vi "PickPlaceAccuracy.vi"() -> ()   [LabVIEW 2019]
panel:
  in  "GoToPlateHB":string="G1 X1143.6066027 Y1005.0612551 F100\rG1 Z64.7125267"
  in  "MatchParameters":T1={"Number of Matches Requested"=1, "Minimum Match Score"=950.0, "Angle Ranges"=[{"Start Angle"=0.0, "End Angle"=0.0}]}
  in  "AtPlate":bool
  in  "SafeMaxZAssembly":dbl=70.0 format="%#_13g"
  in  "Assembly_XYZU":string="G1 X218.5881767 Y999.2858584 F100\rG1 Z67.8627861"
  out "error out":errorcluster
  out "Plate_XYZU":string
  in  "TemplateFileName":string
  out "Image":T2(plugin-control)
  in  "Tolerance":dbl=0.005 format="%#_13g"
  in  "InitialStepSize":dbl=0.1
  in  "SafeMaxZPlate":dbl=77.0 format="%#_13g"
  in  "GoToPlateSi":string="G1 X844.5335768 Y1006.4997118 F100\rG1 Z74.2865084"
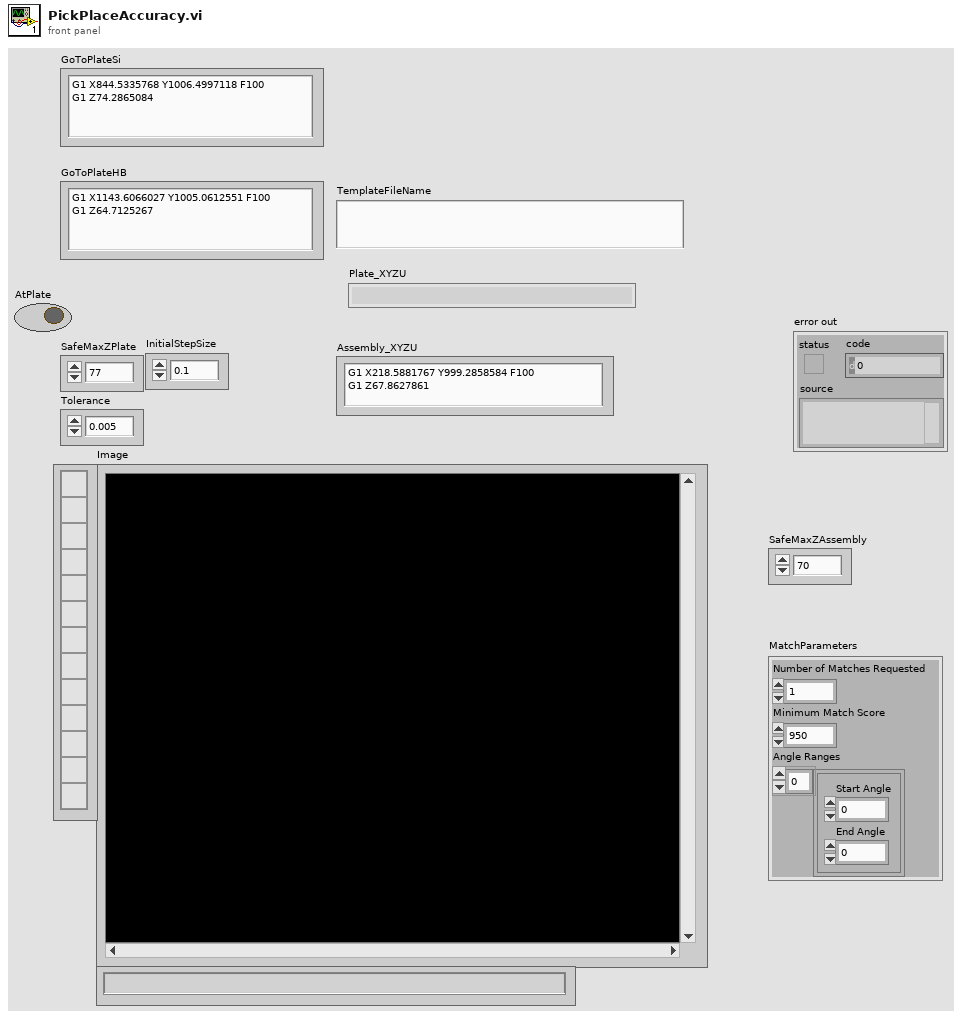
[diagram p1: front panel]
types:
  T1 = cluster{"Number of Matches Requested":i32, "Minimum Match Score":sgl, "Angle Ranges":cluster{"Start Angle":sgl, "End Angle":sgl}[]}
  T2 = typedef "IMAQ Image.ctl" = refnum<image>
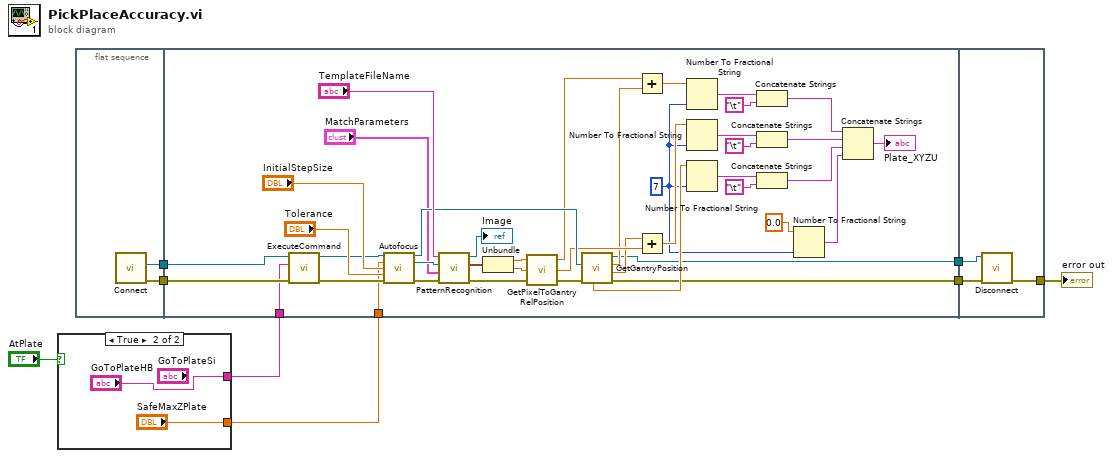
[diagram p0: block diagram]
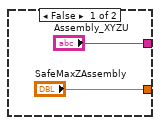
[diagram p2: hidden frame]
diagram:
  n1 = case shown="True" "AtPlate" {
    tunnel: ["Assembly_XYZU" "GoToPlateHB"] -> w4
    tunnel: ["SafeMaxZAssembly" "SafeMaxZPlate"] -> w3
    frame False {
    }
    frame True {
    }
  }
  n2 = flat-sequence {
    tunnel: [w14] -> w8
    tunnel: [w13] -> w6
    tunnel: w8 -> [w54]
    tunnel: w6 -> [w55]
    tunnel: w4 -> [w20]
    tunnel: w3 -> [w19]
    tunnel: [w18] -> w2
    tunnel: [w17] -> w1
    tunnel: [w58] -> w7
    tunnel: w2 -> [w57]
    tunnel: w1 -> [w56]
    frame #0 {
      n3 = call "Connect.vi"() -> ("error out"=w13:errorcluster, "controller"=w14:refnum<k24>)  [unwired: 10 in]
    }
    frame #1 {
      w33 = i16 7 ("precision (6)")
      n4 = call "ExecuteCommand.vi"("error in (no error)"=w55, "Command Code"=w20, "controller in"=w54) -> ("error out"=w21:errorcluster, "controller out"=w22:refnum<k24>)  [unwired: 6 in, 1 out]
      n5 = call "Autofocus.vi"("controller in"=w22, "SafeMaxZ"=w19, "InitialStepSize"="InitialStepSize", "Tolerance"="Tolerance", "error in (no error)"=w21) -> ("controller out"=w50:refnum<k24>, "Image"=w24:T2, "error out"=w29:errorcluster)  [unwired: 6 in, 2 out]
      n6 = call "PatternRecognition.vi"("error in (no error)"=w29, "MatchParameters"="MatchParameters", "ImageIn"=w24, "TemplateFileName"="TemplateFileName") -> ("error out"=w25:errorcluster, "Position"=w28:cluster{"x":sgl, "y":sgl}, "ImageFoundPattern"=→"Image":T2)  [unwired: 2 in, 2 out]
      n7 = Unbundle(w28) -> ("x"=w27:sgl, "y"=w26:sgl)
      n8 = call "GetPixelToGantryRelPosition.vi"("error in (no error)"=w25, "PixelY"=w26, "PixelX"=w27) -> ("error out"=w47:errorcluster, "YmmRelGH"=w48:dbl, "XmmRelGH"=w49:dbl)
      n9 = call "GetGantryPosition.vi"("error in (no error)"=w47, "Controller In"=w50) -> ("error out"=w18:errorcluster, "Position Y"=w36:dbl, "Position X"=w35:dbl, "controller out"=w17:refnum<k24>, "Position Z"=w44:dbl)  [unwired: 3 in, 2 out]
      n10 = Add(x=w49, y=w35) -> (x+y=w42:dbl)
      n11 = Add(x=w36, y=w48) -> (x+y=w43:dbl)
      n12 = Number To Fractional String(number=w42, precision (6)=w33) -> (F-format string=w37:string)  [unwired: 2 in]
      n13 = Number To Fractional String(number=w43, precision (6)=w33) -> (F-format string=w38:string)  [unwired: 2 in]
      n14 = Number To Fractional String(number=w44, precision (6)=w33) -> (F-format string=w45:string)  [unwired: 2 in]
      n15 = Concatenate Strings(w37, "\t") -> (w39:string)
      n16 = Concatenate Strings(w38, "\t") -> (w40:string)
      n17 = Concatenate Strings(w45, "\t") -> (w46:string)
      n18 = Number To Fractional String(number=0.0, precision (6)=w33) -> (F-format string=w16:string)  [unwired: 2 in]
      n19 = Concatenate Strings(w39, w40, w46, w16) -> (→"Plate_XYZU":string)
    }
    frame #2 {
      n20 = call "Disconnect.vi"("error in (no error)"=w57, "controller"=w56) -> ("error out"=w58:errorcluster)  [unwired: 9 in]
    }
  }
  "error out" <- w7
